vi "ExFile5stripGlueNI.vi"() -> ()   [LabVIEW 2010]
panel:
  out "X dim":u32
  out "Y dim":u32
  in  "FileType":u32=67371008
  in  "Calibration ini 2":path
  in  "Upper wavelength":dbl=799.0 format="%.2f"
  in  "Lower wavelength":dbl=239.0 format="%.2f"
  in  "Glue Resolution":dbl=0.1 format="%.2f"
  out "Glue":cluster{"Array":dbl[], "Array F32":sgl[]}(graph)
  in  "Calibration ini":path
  in  "stop":bool
  out "error out":errorcluster
  in  "error in (no error)":errorcluster
  # "ExFile5StripGlueNI : This example takes a calibration file and a data file with 5 strips in a frame. It reads the data file and applies the calibration to it."
  # "Calibration ini file"
  # "Data  file"
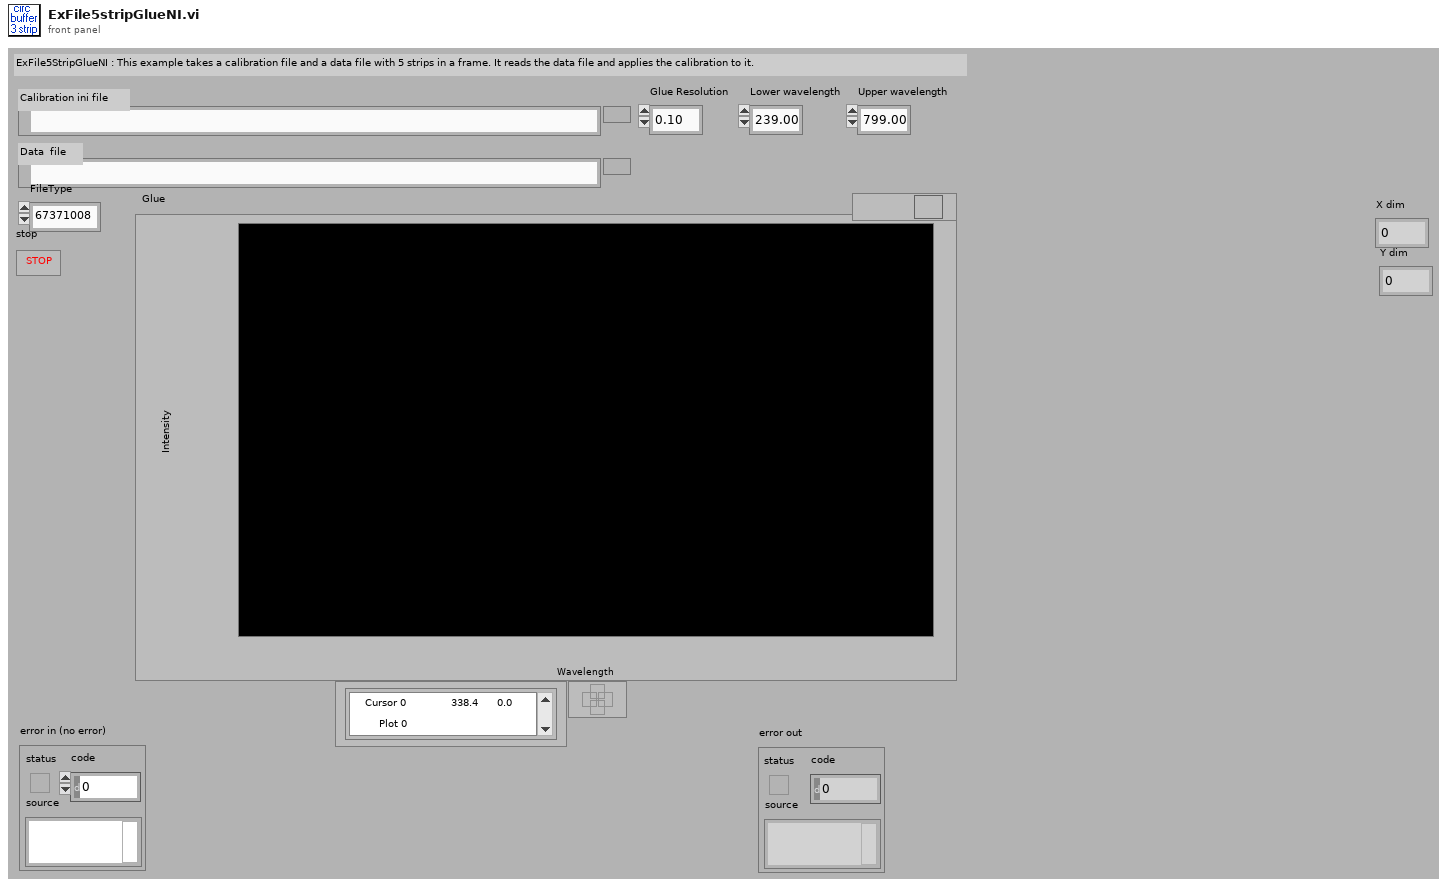
[diagram p1: front panel]
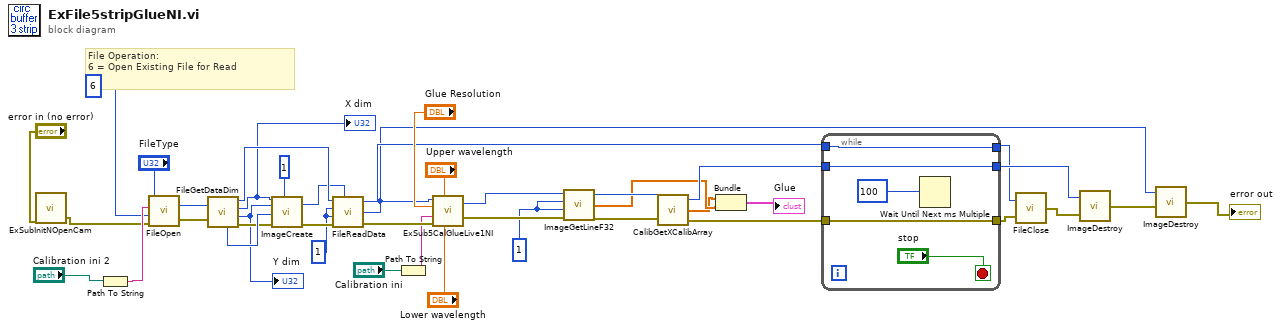
[diagram p0: block diagram]
diagram:
  w16 = 1
  w29 = 1
  # "File Operation:\n6 = Open Existing File for Read"
  n1 = call "ExSubInitNOpenCam.vi"("error in (no error)"="error in (no error)") -> ("error out"=w25:errorcluster)  [unwired: 1 out]
  n2 = Path To String(path="Calibration ini 2") -> (string=w35:string)
  n3 = call <userlib>:"FileOpen.vi"("error in"=w25, "File Operations"=u32 6 ("File Operation"), "FileName"=w35, "File Type"="FileType") -> ("error out"=w38:errorcluster, "File Handle"=w37:u32)
  n4 = call <userlib>:"FileGetDataDim.vi"("File Handle"=w37, "error in"=w38) -> ("Data Type"=w31:u32, "File Handle"=w33:u32, "X dim"=w27:u32, "Y dim"=w28:u32, "error out"=w30:errorcluster)  [unwired: 1 out]
  "X dim" <- w27
  "Y dim" <- w28
  n5 = call <userlib>:"ImageCreate.vi"("X dimension"=w27, "Y dimension"=w28, "Data Type"=w31, "error in"=w30, "Number Of Frames"=1) -> ("Image Handle"=w32:u32, "error out"=w34:errorcluster)
  n6 = call <userlib>:"FileReadData.vi"("File Handle"=w33, "Start Frame"=w29, "End Frame"=w29, "error in"=w34, "Image Handle"=w32) -> ("File Handle"=w8:u32, "Image Handle"=w3:u32, "error out"=w22:errorcluster)
  n7 = Path To String(path="Calibration ini") -> (string=w18:string)
  n8 = call "ExSub5CalGlueLive1NI.vi"("Lower limit"="Lower wavelength", "Upper limit"="Upper wavelength", "error in (no error)"=w22, "String"=w18, "Resolution"="Glue Resolution", "Image Handle"=w3) -> ("error out"=w17:errorcluster, "Glue handle"=w24:u32)
  n9 = call <userlib>:"ImageGetLineF32.vi"("error in"=w17, "Z Position"=w16, "Y Position"=w16, "Data Handle"=w24) -> ("error out"=w15:errorcluster, "Array F32"=w5:sgl[], "Data Handle"=w23:u32)
  n10 = call <userlib>:"CalibGetXCalibArray.vi"("Data Handle"=w23, "error in (no error)"=w15) -> ("Data Handle"=w10:u32, "Array"=w4:dbl[], "error out"=w13:errorcluster)
  n11 = Bundle("Array"=w4, "Array F32"=w5) -> (→"Glue":cluster{"Array":dbl[], "Array F32":sgl[]})  [unwired: 1 in]
  n12 = while {
    tunnel: w13 -> [w46]
    tunnel: [w46] -> w12
    tunnel: w10 -> [w45]
    tunnel: [w45] -> w9
    tunnel: w8 -> [w44]
    tunnel: [w44] -> w7
    stop <- "stop" stop-if-true
    n13 = Wait Until Next ms Multiple(millisecond multiple=100) -> ()  [unwired: 1 out]
  }
  n14 = call <userlib>:"FileClose.vi"("error in"=w12, "File Handle"=w7) -> ("error out"=w11:errorcluster)
  n15 = call <userlib>:"ImageDestroy.vi"("error in"=w11, "Data handle"=w9) -> ("error out"=w2:errorcluster)
  n16 = call <userlib>:"ImageDestroy.vi"("error in"=w2, "Data handle"=w3) -> ("error out"=→"error out":errorcluster)
